vi "RSZVB Set Pulse Modulator.vi"(7 "Pulse Modulator (Off)":bool, 8 "error in (no error)":errorcluster {"code" format="%.0x"}, 9 "Path (1)":i32=1, 10 "Channel (1)":i32=1, 11 "VISA session":refnum<visa-resource-name>) -> (0 "error out":errorcluster {"code" format="%.0x"}, 3 "dup VISA session":refnum<visa-resource-name>)   [LabVIEW 2011]
doc: "This VI loops pulse modulators into the RF signal paths no. <Path>. Paths no. 1 and 3 in the extension unit are source paths, path no. 2 is a receiver path.\n\nRemote-control command(s):\n[SENSe<Ch>:]EUNit:PMODulator<Path>[:STATe]"
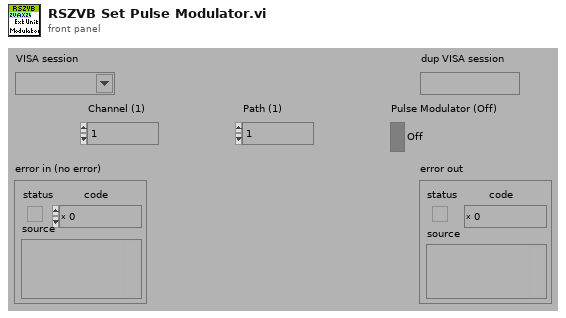
[diagram p1: front panel]
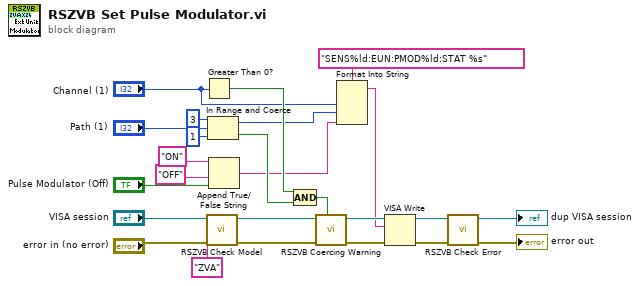
[diagram p0: block diagram]
diagram:
  n1 = Greater Than 0?(x="Channel (1)") -> (x > 0?=w14:bool)
  n2 = call "RSZVB Check Model.vi"("error in (no error)"="error in (no error)", "Model"="ZVA" ("Options"), "VISA session"="VISA session") -> ("error out"=w11:errorcluster, "dup VISA session"=w12:refnum<visa-resource-name>)  [unwired: 7 in]
  n3 = In Range and Coerce(upper limit=3, x="Path (1)", lower limit=1) -> (coerced(x)=w13:i32, In Range?=w15:bool)
  n4 = Append True/False String(1:"Pulse Modulator (Off)", 2:"OFF", 3:"ON") -> (0:w8:string)  [unwired: 1 in]
  n5 = Compound Arithmetic op=AND(w14, w15) -> (w17:bool)
  n6 = call "RSZVB Coercing Warning.vi"("In Range?"=w17, "error in (no error)"=w11, "VISA session"=w12) -> ("error out"=w24:errorcluster, "dup VISA session"=w25:refnum<visa-resource-name>)  [unwired: 7 in]
  n7 = Format Into String(format string="SENS%ld:EUN:PMOD%ld:STAT %s", "Channel (1)", w13, w8) -> (resulting string=w21:string)  [unwired: 2 in, 1 out]
  n8 = VISA Write(VISA resource name=w25, write buffer=w21, error in (no error)=w24) -> (VISA resource name out=w22:refnum<visa-resource-name>, error out=w23:errorcluster)  [unwired: 1 out]
  n9 = call "RSZVB Check Error.vi"("error in (no error)"=w23, "VISA session"=w22) -> ("error out"=→"error out":errorcluster, "dup VISA session"=→"dup VISA session":refnum<visa-resource-name>)  [unwired: 8 in]
